vi "NewComboBox__slk_mt.vi"(8 "error in (no error)":errorcluster, 11 "control refnum in":refnum<vi>) -> (0 "error out":errorcluster, 3 "combobox out":refnum<class "ComboBox__slk_mt.lvclass">)   [LabVIEW 2014, in "Lazyboots Menu Tool.lvlib" / "ComboBox__slk_mt.lvclass"]
doc: "Creates new object of ComboBox class."
uses:
  ComboBox__slk_mt.lvclass
  ComboBox__slk_mt.lvclass/ComboBox__slk_mt.ctl
panel:
  # "NewComboBox__slk_mt.vi\nCreates new object of ComboBox class.\n\nNOTICE -- YOU MUST LEAVE THIS NOTICE IN PLACE.\n\nCopyright (c) 2011, LIANG LIU Shawn.Liu.cn@gmail.com\nAll rights reserved.\n\nRedistribution and use in source and binary forms, with or without modification, are permitted provided that the following conditions are met:\n-Redistributions of source code must retain the above copyright notice, this list of conditions and the following disclaimer.\n-Redistributions in binary form must reproduce the above copyright notice, this list of conditions and the following disclaimer in the documentation and/or other materials provided with the distribution.\n-Neither the name of the eLp nor the names of its contributors may be used to endorse or promote products derived from this software without specific prior written permission.\n\nTHIS SOFTWARE IS PROVIDED BY THE COPYRIGHT HOLDERS AND CONTRIBUTORS \"AS IS\" AND ANY EXPRESS OR IMPLIED WARRANTIES, INCLUDING, BUT NOT LIMITED TO, THE IMPLIED WARRANTIES OF MERCHANTABILITY AND FITNESS FOR A PARTICULAR PURPOSE ARE DISCLAIMED. IN NO EVENT SHALL THE COPYRIGHT HOLDER OR CONTRIBUTORS BE LIABLE FOR ANY DIRECT, INDIRECT, INCIDENTAL, SPECIAL, EXEMPLARY, OR CONSEQUENTIAL DAMAGES (INCLUDING, BUT NOT LIMITED TO, PROCUREMENT OF SUBSTITUTE GOODS OR SERVICES; LOSS OF USE, DATA, OR PROFITS; OR BUSINESS INTERRUPTION) HOWEVER CAUSED AND ON ANY THEORY OF LIABILITY, WHETHER IN CONTRACT, STRICT LIABILITY, OR TORT (INCLUDING NEGLIGENCE OR OTHERWISE) ARISING IN ANY WAY OUT OF THE USE OF THIS SOFTWARE, EVEN IF ADVISED OF THE POSSIBILITY OF SUCH DAMAGE."
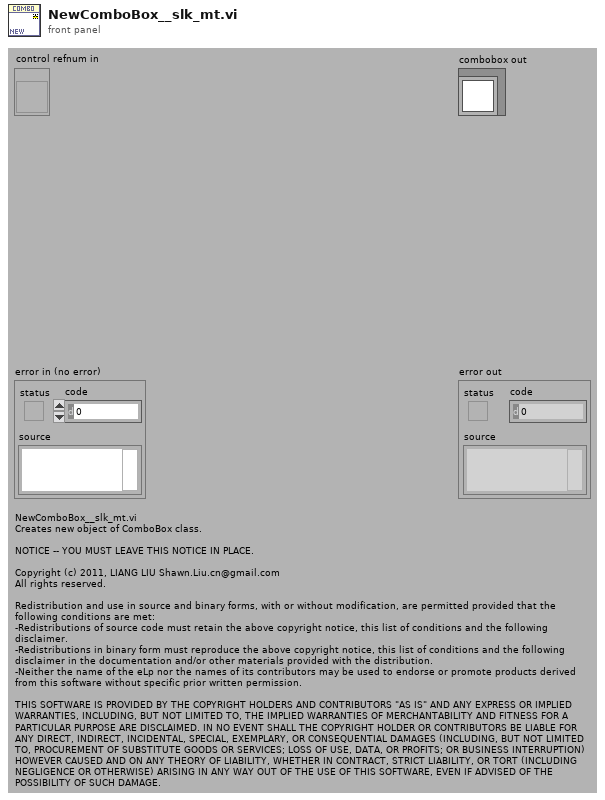
[diagram p1: front panel]
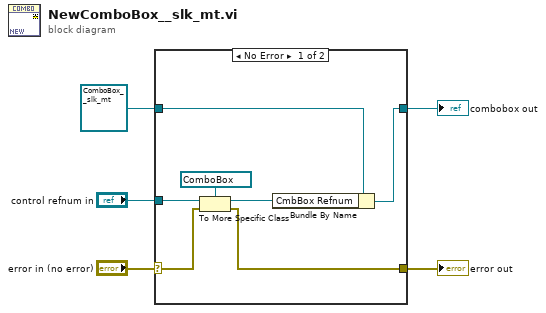
[diagram p0: block diagram]
diagram:
  n1 = case shown="No Error" "error in (no error)" {
    selector: "error in (no error)" -> [w9 w14]
    tunnel: [w8 w14] -> w4
    tunnel: [w6 w13] -> w2
    tunnel: refnum<class "ComboBox__slk_mt.lvclass"> refnum ("combobox__slk_mt in") -> [w7 w13]
    tunnel: "control refnum in" -> [w12 _]
    frame No Error {
      n2 = To More Specific Class(target class=refnum<vi> refnum ("CmbBox Refnum"), reference=w12, error in=w9) -> (specific class reference=w11:refnum<vi>, error out=w8:errorcluster)
      n3 = Bundle By Name(cluster=w7, "CmbBox Refnum"=w11) -> (w6:refnum<class "ComboBox__slk_mt.lvclass">)
    }
    frame Error {
    }
  }
  "error out" <- w4
  "combobox out" <- w2
